vi "Enqueue Send Frames.vi"(0 "ZCAN_Transmit_Data":T2, 1 "Protocol":u32(ring)=1 items=["CAN", "CANFD"], 3 "ChannelHandle":u32, 5 "ZCAN_TransmitFD_Data":T1, 7 "Frames":u32, 12 "Timestamp":timestamp) -> ()   [LabVIEW 2011, in "CAN FD.lvlib"]
uses:
  CAN FD.lvlib
  data_type/ZCAN_Transmit_Data.ctl
  data_type/ZCAN_TransmitFD_Data.ctl
  Typedef/CAN Data.ctl
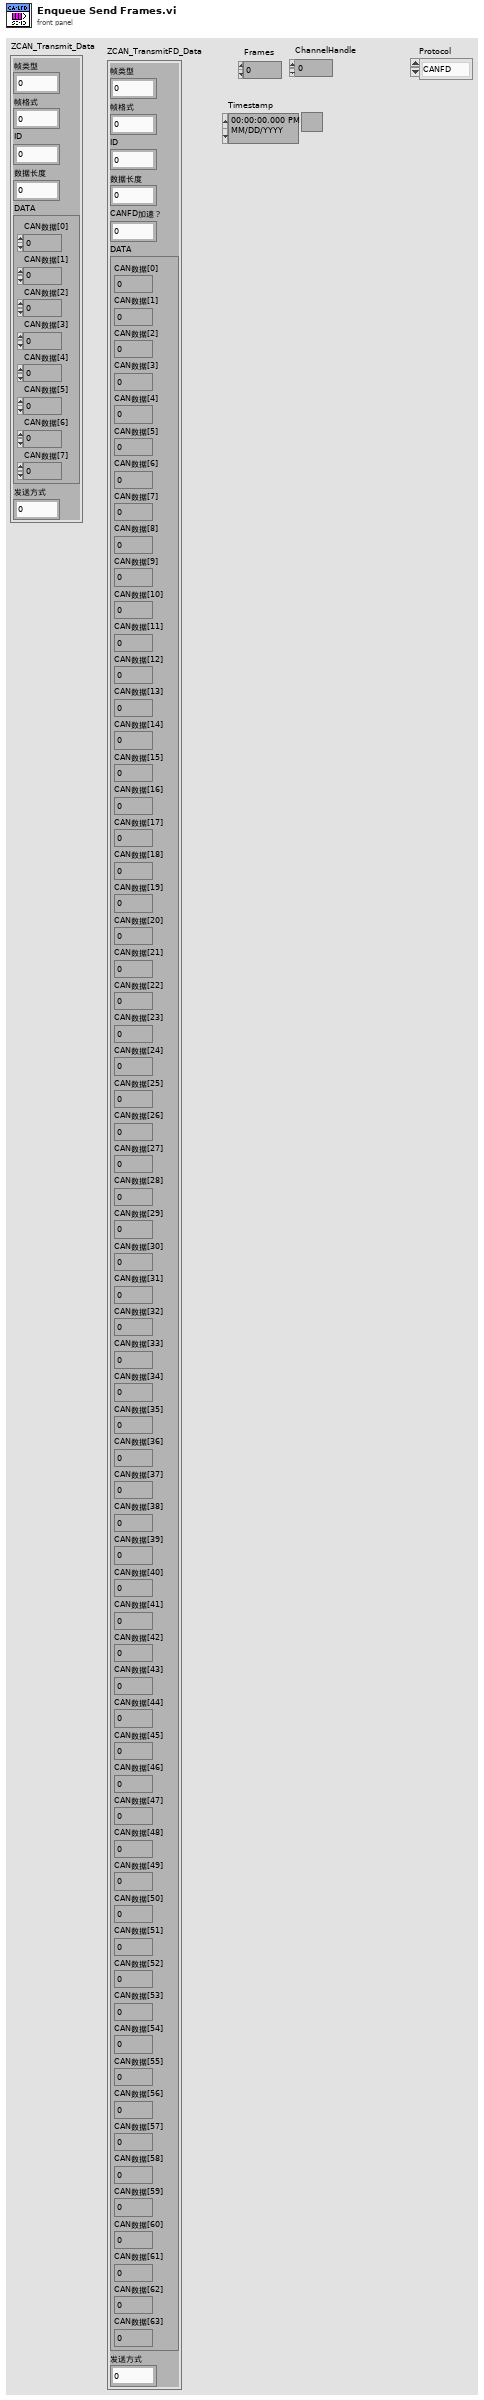
[diagram p1: front panel]
types:
  T1 = typedef "ZCAN_TransmitFD_Data.ctl" = cluster{"帧类型":u32, "帧格式":u32, "ID":u32, "数据长度":u8, "CANFD加速？":u8, "DATA":cluster{"CAN数据[0]":u8, "CAN数据[1]":u8, "CAN数据[2]":u8, "CAN数据[3]":u8, "CAN数据[4]":u8, "CAN数据[5]":u8, "CAN数据[6]":u8, "CAN数据[7]":u8, "CAN数据[8]":u8, "CAN数据[9]":u8, "CAN数据[10]":u8, "CAN数据[11] ":u8, "CAN数据[12] ":u8, "CAN数据[13] ":u8, "CAN数据[14] ":u8, "CAN数据[15] ":u8, "CAN数据[16]":u8, "CAN数据[17]":u8, "CAN数据[18]":u8, "CAN数据[19]":u8, "CAN数据[20]":u8, "CAN数据[21]":u8, "CAN数据[22]":u8, "CAN数据[23]":u8, "CAN数据[24] ":u8, "CAN数据[25]":u8, "CAN数据[26]":u8, "CAN数据[27]":u8, "CAN数据[28]":u8, "CAN数据[29]":u8, "CAN数据[30]":u8, "CAN数据[31]":u8, "CAN数据[32]":u8, "CAN数据[33]":u8, "CAN数据[34]":u8, "CAN数据[35]":u8, "CAN数据[36]":u8, "CAN数据[37]":u8, "CAN数据[38]":u8, "CAN数据[39]":u8, "CAN数据[40]":u8, "CAN数据[41]":u8, "CAN数据[42]":u8, "CAN数据[43]":u8, "CAN数据[44]":u8, "CAN数据[45]":u8, "CAN数据[46]":u8, "CAN数据[47]":u8, "CAN数据[48]":u8, "CAN数据[49]":u8, "CAN数据[50]":u8, "CAN数据[51]":u8, "CAN数据[52]":u8, "CAN数据[53]":u8, "CAN数据[54]":u8, "CAN数据[55]":u8, "CAN数据[56]":u8, "CAN数据[57]":u8, "CAN数据[58]":u8, "CAN数据[59]":u8, "CAN数据[60]":u8, "CAN数据[61]":u8, "CAN数据[62]":u8, "CAN数据[63]":u8}, "发送方式":u32}
  T2 = typedef "ZCAN_Transmit_Data.ctl" = cluster{"帧类型":u32, "帧格式":u32, "ID":u32, "数据长度":u8, "DATA":cluster{"CAN数据[0]":u8, "CAN数据[1]":u8, "CAN数据[2]":u8, "CAN数据[3]":u8, "CAN数据[4]":u8, "CAN数据[5]":u8, "CAN数据[6]":u8, "CAN数据[7]":u8}, "发送方式":u32}
  T3 = typedef "CAN FD.lvlib/CAN Data.ctl" = cluster{"SystemTime":timestamp, "HwTime":dbl, "Channel":u8, "ID":u32, "CANType":i16, "Direction":i16, "Remote":bool, "Ext":bool, "Len":u8, "Data":u8[], "Success":bool}
  T4 = cluster{"CAN数据[0]":u8, "CAN数据[1]":u8, "CAN数据[2]":u8, "CAN数据[3]":u8, "CAN数据[4]":u8, "CAN数据[5]":u8, "CAN数据[6]":u8, "CAN数据[7]":u8}
  T5 = cluster{"CAN数据[0]":u8, "CAN数据[1]":u8, "CAN数据[2]":u8, "CAN数据[3]":u8, "CAN数据[4]":u8, "CAN数据[5]":u8, "CAN数据[6]":u8, "CAN数据[7]":u8, "CAN数据[8]":u8, "CAN数据[9]":u8, "CAN数据[10]":u8, "CAN数据[11] ":u8, "CAN数据[12] ":u8, "CAN数据[13] ":u8, "CAN数据[14] ":u8, "CAN数据[15] ":u8, "CAN数据[16]":u8, "CAN数据[17]":u8, "CAN数据[18]":u8, "CAN数据[19]":u8, "CAN数据[20]":u8, "CAN数据[21]":u8, "CAN数据[22]":u8, "CAN数据[23]":u8, "CAN数据[24] ":u8, "CAN数据[25]":u8, "CAN数据[26]":u8, "CAN数据[27]":u8, "CAN数据[28]":u8, "CAN数据[29]":u8, "CAN数据[30]":u8, "CAN数据[31]":u8, "CAN数据[32]":u8, "CAN数据[33]":u8, "CAN数据[34]":u8, "CAN数据[35]":u8, "CAN数据[36]":u8, "CAN数据[37]":u8, "CAN数据[38]":u8, "CAN数据[39]":u8, "CAN数据[40]":u8, "CAN数据[41]":u8, "CAN数据[42]":u8, "CAN数据[43]":u8, "CAN数据[44]":u8, "CAN数据[45]":u8, "CAN数据[46]":u8, "CAN数据[47]":u8, "CAN数据[48]":u8, "CAN数据[49]":u8, "CAN数据[50]":u8, "CAN数据[51]":u8, "CAN数据[52]":u8, "CAN数据[53]":u8, "CAN数据[54]":u8, "CAN数据[55]":u8, "CAN数据[56]":u8, "CAN数据[57]":u8, "CAN数据[58]":u8, "CAN数据[59]":u8, "CAN数据[60]":u8, "CAN数据[61]":u8, "CAN数据[62]":u8, "CAN数据[63]":u8}
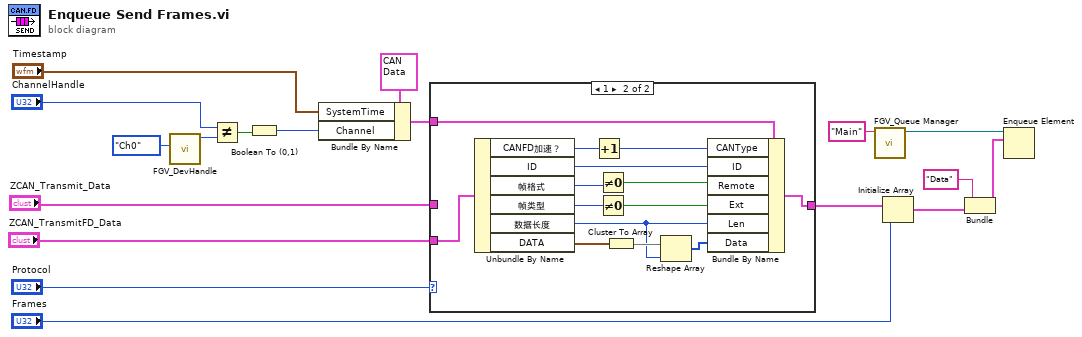
[diagram p0: block diagram]
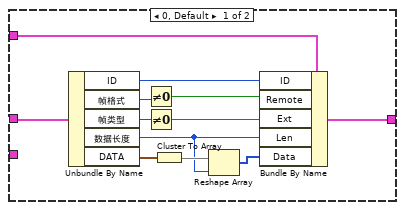
[diagram p2: hidden frame]
diagram:
  n1 = call "FGV_DevHandle.vi"("Type"=enum16{"Device", "Ch0", "Ch1"}."Ch0") -> ("handle out"=w9:u32)  [unwired: 8 in, 2 out]
  n2 = Not Equal?(x="ChannelHandle", y=w9) -> (x != y?=w8:bool)
  n3 = Boolean To (0,1)(Boolean=w8) -> (0, 1=w7:i16)
  n4 = Bundle By Name(cluster=T3 {"SystemTime"=timestamp(0 s since 1904-01-01), "HwTime"=0.0, "Channel"=0, "ID"=0, "CANType"=0, "Direction"=0, "Remote"=FALSE, "Ext"=FALSE, "Len"=0, "Data"=[], "Success"=FALSE} ("Data"), "SystemTime"="Timestamp", "Channel"=w7) -> (w11:T3)
  n5 = case shown="1" "Protocol" {
    tunnel: "ZCAN_Transmit_Data" -> [w19 _]
    tunnel: w11 -> [w30 w44]
    tunnel: [w20 w34] -> w6
    tunnel: "ZCAN_TransmitFD_Data" -> [_ w31]
    frame 0, Default {
      n6 = Unbundle By Name(w19) -> ("ID"=w29:u32, "帧格式"=w27:u32, "帧类型"=w28:u32, "数据长度"=w22:u8, "DATA"=w24:T4)
      n7 = Not Equal To 0?(x=w27) -> (x != 0?=w26:bool)
      n8 = Not Equal To 0?(x=w28) -> (x != 0?=w25:bool)
      n9 = Cluster To Array(cluster=w24) -> (array=w23:u8[])
      n10 = Reshape Array(w23, w22) -> (w21:u8[])
      n11 = Bundle By Name(cluster=w30, "ID"=w29, "Remote"=w26, "Ext"=w25, "Len"=w22, "Data"=w21) -> (w20:T3)
    }
    frame 1 {
      n12 = Unbundle By Name(w31) -> ("CANFD加速？"=w33:u8, "ID"=w43:u32, "帧格式"=w41:u32, "帧类型"=w42:u32, "数据长度"=w36:u8, "DATA"=w38:T5)
      n13 = Increment(x=w33) -> (x+1=w32:u8)
      n14 = Not Equal To 0?(x=w41) -> (x != 0?=w40:bool)
      n15 = Not Equal To 0?(x=w42) -> (x != 0?=w39:bool)
      n16 = Cluster To Array(cluster=w38) -> (array=w37:u8[])
      n17 = Reshape Array(w37, w36) -> (w35:u8[])
      n18 = Bundle By Name(cluster=w44, "CANType"=w32, "ID"=w43, "Remote"=w40, "Ext"=w39, "Len"=w36, "Data"=w35) -> (w34:T3)
    }
  }
  n19 = call "FGV_Queue Manager.vi"("Name"="Main") -> ("Queue"=w5:refnum<queue>)  [unwired: 8 in, 2 out]
  n20 = Initialize Array(w6, "Frames") -> (w4:T3[])
  n21 = Bundle("Data", w4) -> (w2:cluster{string, T3[]})  [unwired: 1 in]
  n22 = Enqueue Element(queue=w5, element=w2) -> ()  [unwired: 2 in, 3 out]
